vi "NanoCorrelation.vi"(7 "Simple Thresh Count?":bool, 9 "Cluster":T1={"dB Thresh"=0.0, "Mask Start"=4, "Mask length"=0}, 10 "Array":dbl[][](array[numeric]), 11 "Previous Agent Indexes":u8[](array[numeric])) -> (0 "max correlation shift":i32, 1 "Agent Indexes":u8[](array[numeric]), 2 "Rxy":dbl[](array[numeric]), 3 "New Count":i16, 4 "Max dB out":dbl, 5 "RF Trace":dbl[][](array[numeric]), 6 "Max in Window":dbl[](array[numeric]))   [LabVIEW 2022 SP3]
uses:
  <vilib>/Analysis/2dsp.llb/1D Cross Correlation (DBL).vi
  <vilib>/Analysis/NI_AALPro.lvlib
panel:
  out "Binary n and n+1 frame":i16[][](graph)
  out "Correlation Graph":dbl[](graph)
  out "Raw data":dbl[][](graph)
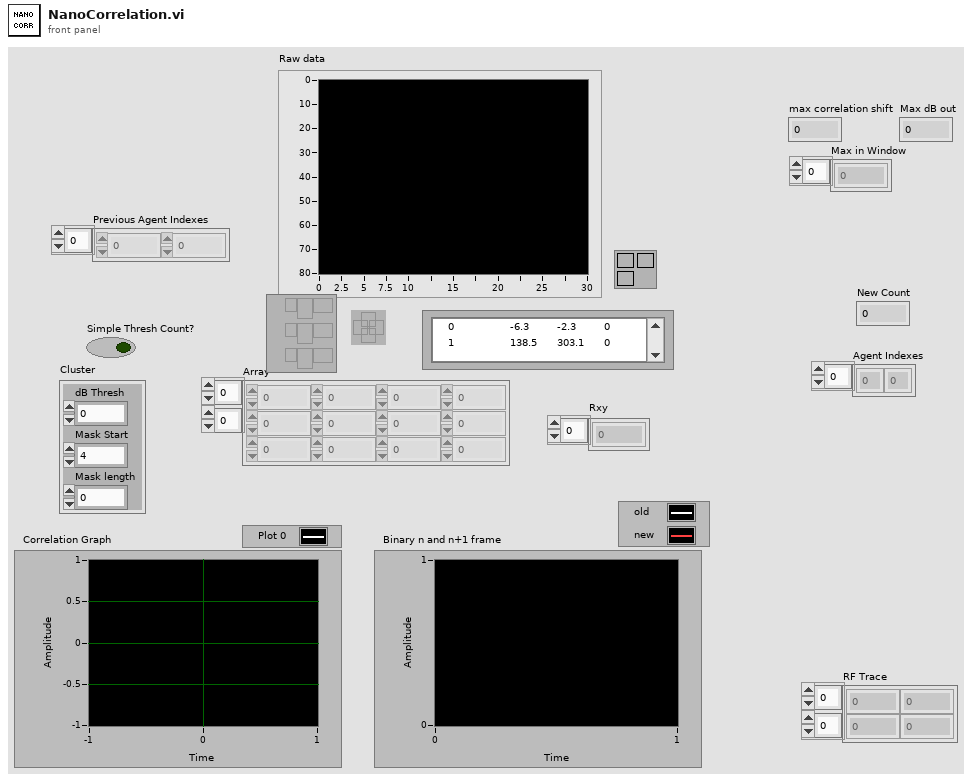
[diagram p1: front panel]
types:
  T1 = cluster{"dB Thresh":dbl, "Mask Start":i32, "Mask length":i32}
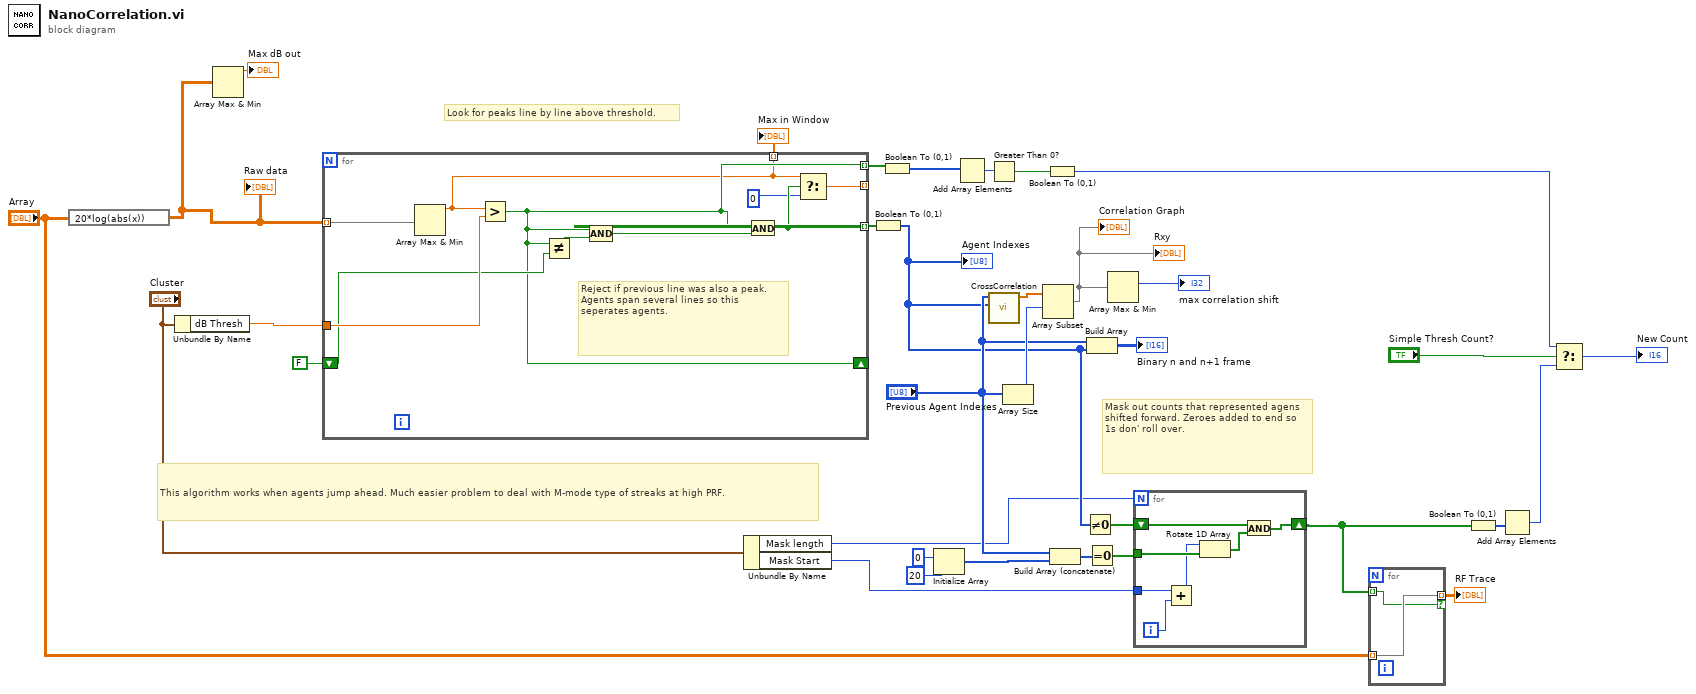
[diagram p0: block diagram]
diagram:
  # "This algorithm works when agents jump ahead. Much easier problem to deal with M-mode type of streaks at high PRF."
  # "Mask out counts that represented agens shifted forward. Zeroes added to end so 1s don' roll over."
  # "Look for peaks line by line above threshold."
  n1 = expression code="20*log(abs(x))"("Array") -> (w2:dbl[][])
  "Raw data" <- w2
  n2 = Unbundle By Name("Cluster") -> ("dB Thresh"=w17:dbl)
  n3 = Array Max & Min(array=w2) -> (max value=→"Max dB out":dbl)  [unwired: 3 out]
  n4 = for {
    tunnel: w2 -> [w35] mode=indexing
    tunnel: [w40] -> w33 mode=indexing
    tunnel: w17 -> [w44]
    shift-right: [w37] -> _
    shift-left: FALSE -> [w43]
    tunnel: [w38] -> _ mode=indexing
    tunnel: [w37] -> w10 mode=indexing
    tunnel: [w36] -> w1 mode=indexing
    # "Reject if previous line was also a peak. Agents span several lines so this seperates agents."
    n5 = Array Max & Min(array=w35) -> (max value=w36:dbl)  [unwired: 3 out]
    n6 = Greater?(x=w36, y=w44) -> (0:w37:bool)
    n7 = Not Equal?(x=w37, y=w43) -> (x != y?=w42:bool)
    n8 = Compound Arithmetic op=AND(w37, w42) -> (w41:bool)
    n9 = And(x=w37, y=w41) -> (x .and. y?=w40:bool)
    n10 = Select(t=w36, s=w40, f=0) -> (s? t:f=w38:dbl)
  }
  "Max in Window" <- w1
  n11 = Unbundle By Name("Cluster") -> ("Mask length"=w15:i32, "Mask Start"=w14:i32)
  n12 = Boolean To (0,1)(Boolean=w33) -> (0, 1=w25:i16[])
  "Agent Indexes" <- w25
  n13 = Boolean To (0,1)(Boolean=w10) -> (0, 1=w9:i16[])
  n14 = Initialize Array(0 ("element"), 20 ("dimension size")) -> (w27:i32[])
  n15 = Add Array Elements(numeric array=w9) -> (sum=w8:i16)
  n16 = Greater Than 0?(x=w8) -> (x > 0?=w7:bool)
  n17 = call-poly <vilib>:"CrossCorrelation.vi"("Y"=w25, "X"="Previous Agent Indexes") -> ("Rxy"=w31:dbl[])  [unwired: 8 in, 1 out]
  n18 = Array Size(array="Previous Agent Indexes") -> (size(s)=w30:i32)
  n19 = Array Subset(array=w31, index=w30) -> (w20:dbl[])  [unwired: 1 in]
  "Rxy" <- w20
  "Correlation Graph" <- w20
  n20 = Boolean To (0,1)(Boolean=w7) -> (0, 1=w6:i16)
  n21 = Build Array (concatenate)("Previous Agent Indexes", w27) -> (w24:i32[])
  n22 = Not Equal To 0?(x=w25) -> (x != 0?=w21:bool[])
  n23 = Build Array("Previous Agent Indexes", w25) -> (→"Binary n and n+1 frame":i16[][])
  n24 = Equal To 0?(x=w24) -> (x = 0?=w22:bool[])
  n25 = Array Max & Min(array=w20) -> (max index (indices)=→"max correlation shift":i32)  [unwired: 3 out]
  n26 = for {
    N: w15 -> [_]
    shift-right: [w50] -> w13
    shift-left: w21 -> [w51]
    tunnel: w14 -> [w48]
    tunnel: w22 -> [w47]
    i -> [w49]
    n27 = Add(x=w48, y=w49) -> (x+y=w46:i32)
    n28 = Rotate 1D Array(1:w47, 2:w46) -> (0:w45:bool[])
    n29 = And(x=w51, y=w45) -> (x .and. y?=w50:bool[])
  }
  n30 = for {
    tunnel: w13 -> [w52] mode=indexing
    tunnel: "Array" -> [w53] mode=indexing
    tunnel: [w53] -> w12 mode=indexing if=w52
  }
  "RF Trace" <- w12
  n31 = Boolean To (0,1)(Boolean=w13) -> (0, 1=w23:i16[])
  n32 = Add Array Elements(numeric array=w23) -> (sum=w5:i16)
  n33 = Select(t=w6, s="Simple Thresh Count?", f=w5) -> (s? t:f=→"New Count":i16)
